vi "Collide.vi"(9 "Team in":refnum<class "Team.lvclass">, 11 "MySquare in":refnum<class "MySquare.lvclass">) -> (1 "Team out":refnum<class "Team.lvclass">, 3 "MySquare out":refnum<class "MySquare.lvclass">)   [LabVIEW 2020, in "Clones.lvlib" / "MySquare.lvclass"]
uses:
  MySquare.lvclass
  SquareBattle/Team/Team.lvclass
  MyTeam/MyTeam.lvclass
  C:/Apps/GIE/Instructions Test/SquareBattle/Team/Team.lvclass
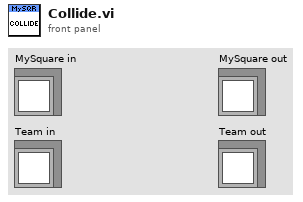
[diagram p1: front panel]
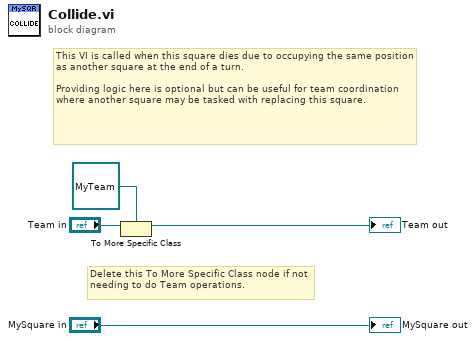
[diagram p0: block diagram]
diagram:
  # "Delete this To More Specific Class node if not needing to do Team operations."
  # "This VI is called when this square dies due to occupying the same position as another square at the end of a turn.\n\nProviding logic here is optional but can be useful for team coordination where another square may be tasked with replacing this square."
  n1 = To More Specific Class(target class=refnum<class "MyTeam.lvclass"> refnum ("SquareTeam.lvlib:MyTeam.lvclass"), reference="Team in") -> (specific class reference=→"Team out":refnum<class "MyTeam.lvclass">)  [unwired: 1 in, 1 out]
  "MySquare out" <- "MySquare in"
